vi "Init.vi"(0 "Serial 输入":refnum<class "Serial.lvclass"> caption="DNL_LabVIEW Object in", 5 "控制端口":refnum<visa-resource-name>, 7 "波特率":u32, 9 "ReadDelay":u32, 11 "error in (no error)":errorcluster caption="错误输入（无错误）") -> (4 "Serial 输出":refnum<class "Serial.lvclass"> caption="DNL_LabVIEW Object out", 15 "error out":errorcluster caption="错误输出")   [LabVIEW 2012, in "Serial.lvclass"]
uses:
  Serial.lvclass
  PComm/PCOMM.lvlib
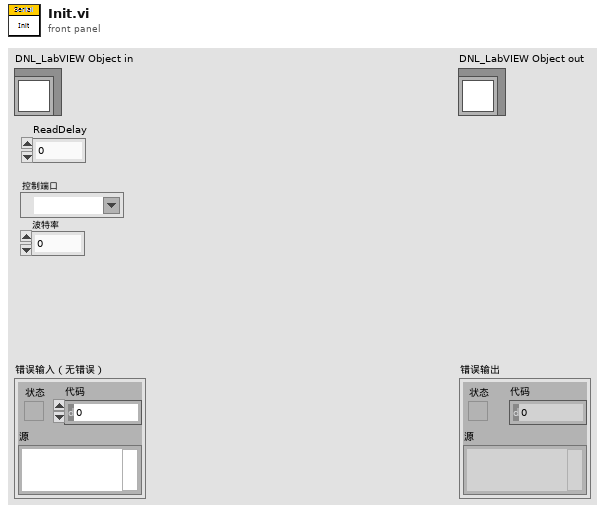
[diagram p1: front panel]
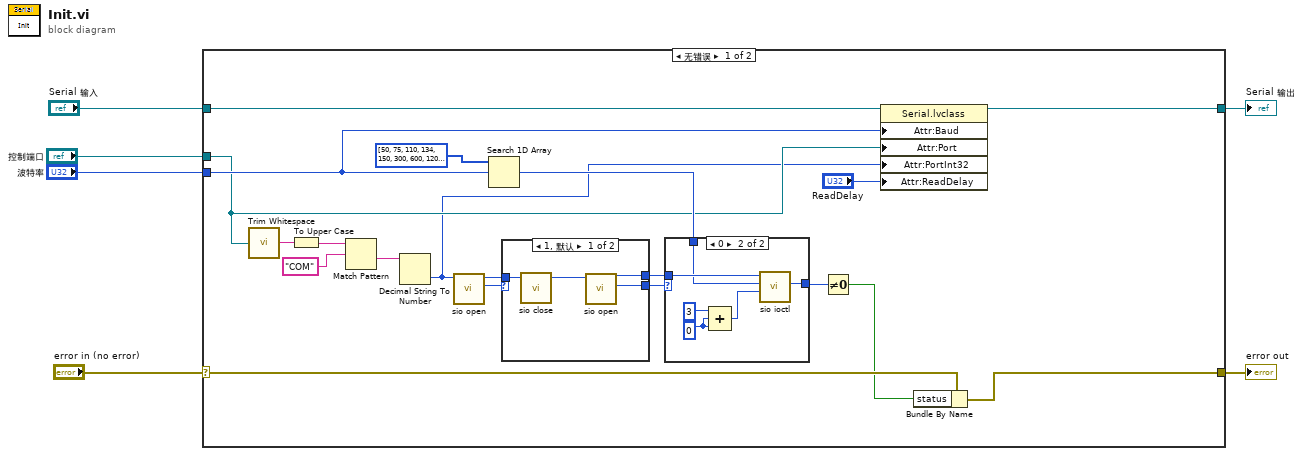
[diagram p0: block diagram]
diagram:
  n1 = case shown="无错误" "error in (no error)" {
    selector: "error in (no error)" -> [w10 w41]
    tunnel: [w8 w41] -> w5
    tunnel: [w13 w40] -> w3
    tunnel: "Serial 输入" -> [w16 w40]
    tunnel: "控制端口" -> [w14 _]
    tunnel: "波特率" -> [w15 _]
    frame No Error {
      n2 = call <vilib>:"Trim Whitespace.vi"("string"=w14) -> ("trimmed string"=w26:string)  [unwired: 1 in]
      n3 = To Upper Case(1:w26) -> (0:w25:string)
      n4 = Match Pattern(string=w25, regular expression="COM" ("正则表达式")) -> (after substring=w23:string)  [unwired: 1 in, 3 out]
      n5 = Decimal String To Number(string=w23) -> (number=w12:i32)  [unwired: 2 in, 1 out]
      n6 = call "sio open.vi"("port"=w12) -> ("function return"=w21:i32, "port"=w20:i32)  [unwired: 8 in]
      n7 = Search 1D Array(1D array=i32[] [50, 75, 110, 134, 150, 300, 600, 1200, 1800, 2400, 4800, 7200, 9600, 19200, 38400, 57600, 115200, 230400, 460800, 921600], element=w15) -> (index of element=w17:i32)  [unwired: 1 in]
      n8 = case shown="1, 默认" w21 {
        selector: w21 -> [_ w39]
        tunnel: [w37 w39] -> w22
        tunnel: w20 -> [w36 w38]
        tunnel: [w34 w38] -> w19
        frame 1, Default {
          n9 = call "sio close.vi"("port"=w36) -> ("port"=w35:i32)  [unwired: 8 in, 1 out]
          n10 = call "sio open.vi"("port"=w35) -> ("function return"=w37:i32, "port"=w34:i32)  [unwired: 8 in]
        }
        frame 0 {
        }
      }
      n11 = case shown="0" w22 {
        selector: w22 -> [w27 _]
        tunnel: [w27 w30] -> w11
        tunnel: w19 -> [_ w29]
        tunnel: w17 -> [_ w28]
        frame -1, Default {
        }
        frame 0 {
          w31 = 0
          n12 = Compound Arithmetic op=unknown(3, w31, w31) -> (w33:i32)
          n13 = call "sio ioctl.vi"("mode"=w33, "baud"=w28, "port"=w29) -> ("function return"=w30:i32)  [unwired: 6 in, 1 out]
        }
      }
      n14 = Not Equal To 0?(x=w11) -> (x != 0?=w9:bool)
      n15 = property class="Serial.lvclass"(reference=w16, "Attr:Baud"=w15, "Attr:Port"=w14, "Attr:PortInt32"=w12, "Attr:ReadDelay"="ReadDelay") -> (reference out=w13:refnum<class "Serial.lvclass">)  [unwired: 1 in, 1 out]
      n16 = Bundle By Name(cluster=w10, "status"=w9) -> (w8:errorcluster)
    }
    frame Error {
    }
  }
  "error out" <- w5
  "Serial 输出" <- w3
